vi "DAQ_olfactometer_control.vi"() -> ()   [LabVIEW 2016]
uses:
  <vilib>/DAQmx/write.llb/DAQmx Write (Digital 1D Wfm NChan NSamp).vi
  <vilib>/DAQmx/read.llb/DAQmx Read (Analog 1D Wfm NChan NSamp).vi
  <vilib>/Waveform/DWDTOps.llb/DWDT Uncompress Digital.vi
  <vilib>/DAQmx/miscellaneous.llb/DAQmx Fill In Error Info.vi
panel:
  out "flows":waveform(dbl)[](graph)
  in  "Analog input sampling time (s)":dbl=2.0 format="%#_13g"
  in  "Odour bottles":T1(array[cluster])=[[{"Mixture components"=[{"Name"="MINERAL OIL", "CID"=0, "Volatility"=0.0}], "Name"="B1 (Bl)", "VPs"="0.0E+0", "Proportion"=[{"Numeric"=100.0}], "Selected"=FALSE, "Counter"=TRUE}, {"Mixture components"=[{"Name"="Methyl benzoate", "CID"=8103, "Volatility"=0.38}, {"Name"="Menthone", "CID"=8063, "Volatility"=0.28}], "Name"="B3 (ME2)", "VPs"="3.3E-1 ± 21%", "Proportion"=[{"Numeric"=50.0}, {"Numeric"=50.0}], "Selected"=TRUE, "Counter"=FALSE}, {"Mixture components"=[{"Name"="Decanol", "CID"=460, "Volatility"=0.00851}], "Name"="B5 (C4f)", "VPs"="8.5E-3", "Proportion"=[{"Numeric"=100.0}], "Selected"=FALSE, "Counter"=FALSE}, {"Mixture components"=[{"Name"="Acetophenone", "CID"=8174, "Volatility"=0.45}, {"Name"="Fenchone", "CID"=8635, "Volatility"=0.82}], "Name"="B7 (ME1)", "VPs"="6.4E-1 ± 41%", "Proportion"=[{"Numeric"=50.0}, {"Numeric"=50.0}], "Selected"=FALSE, "Counter"=FALSE}], [{"Mixture components"=[{"Name"="MINERAL OIL", "CID"=0, "Volatility"=0.0}], "Name"="B2 (Bl)", "VPs"="0.0E+0", "Proportion"=[{"Numeric"=100.0}], "Selected"=FALSE, "Counter"=TRUE}, {"Mixture components"=[{"Name"="Octanol", "CID"=7439, "Volatility"=0.0794}], "Name"="B4 (C4cA)", "VPs"="7.9E-2", "Proportion"=[{"Numeric"=100.0}], "Selected"=FALSE, "Counter"=FALSE}, {"Mixture components"=[{"Name"="MINERAL OIL", "CID"=0, "Volatility"=0.0}], "Name"="B6 (Bl)", "VPs"="0.0E+0", "Proportion"=[{"Numeric"=100.0}], "Selected"=FALSE, "Counter"=FALSE}, {"Mixture components"=[{"Name"="Heptanoic acid ", "CID"=957, "Volatility"=0.0107}], "Name"="B8 (C3cA)", "VPs"="1.1E-2", "Proportion"=[{"Numeric"=100.0}], "Selected"=FALSE, "Counter"=FALSE}], [{"Mixture components"=[{"Name"="MINERAL OIL", "CID"=0, "Volatility"=0.0}], "Name"="B9 (Bl)", "VPs"="0.0E+0", "Proportion"=[{"Numeric"=100.0}], "Selected"=FALSE, "Counter"=TRUE}, {"Mixture components"=[{"Name"="Geranyl acetate", "CID"=6985, "Volatility"=0.03}, {"Name"="Dimethylacetophenone", "CID"=7144, "Volatility"=0.063}], "Name"="B11 (MW1)", "VPs"="4.6E-2 ± 50%", "Proportion"=[{"Numeric"=50.0}, {"Numeric"=50.0}], "Selected"=FALSE, "Counter"=FALSE}, {"Mixture components"=[{"Name"="Geraniol", "CID"=6405, "Volatility"=0.03}, {"Name"="Phenyl butanone", "CID"=7762, "Volatility"=0.1}], "Name"="B13 (MW2)", "VPs"="6.5E-2 ± 76%", "Proportion"=[{"Numeric"=50.0}, {"Numeric"=50.0}], "Selected"=FALSE, "Counter"=FALSE}, {"Mixture components"=[{"Name"="Methylheptanoic acid", "CID"=1032, "Volatility"=0.018}], "Name"="B15 (C3f)", "VPs"="1.8E-2", "Proportion"=[{"Numeric"=100.0}], "Selected"=FALSE, "Counter"=FALSE}], [{"Mixture components"=[{"Name"="MINERAL OIL", "CID"=0, "Volatility"=0.0}], "Name"="B10 (Bl)", "VPs"="0.0E+0", "Proportion"=[{"Numeric"=100.0}], "Selected"=FALSE, "Counter"=FALSE}, {"Mixture components"=[{"Name"="Valeric acid", "CID"=8025, "Volatility"=0.196}], "Name"="B12 (C3cB)", "VPs"="2.0E-1", "Proportion"=[{"Numeric"=100.0}], "Selected"=FALSE, "Counter"=FALSE}, {"Mixture components"=[{"Name"="Nonanol", "CID"=4133, "Volatility"=0.0227}], "Name"="B14 (C4cB)", "VPs"="2.3E-2", "Proportion"=[{"Numeric"=100.0}], "Selected"=FALSE, "Counter"=FALSE}, {"Mixture components"=[{"Name"="Hydroxacetophenone", "CID"=7462, "Volatility"=0.0856}], "Name"="B16 (Ol)", "VPs"="8.6E-2", "Proportion"=[{"Numeric"=100.0}], "Selected"=FALSE, "Counter"=FALSE}]]
  in  "Olfactometer parameters":T2={"Back valve ON delays"=[0.0, 0.0, 0.0, 0.0, 0.0, 0.0, 0.0, 0.0, 0.0, 0.0, 0.0, 0.0, 0.0, 0.0, 0.0, 0.0], "Back valve OFF delays"=[0.0, 0.0, 0.0, 0.0, 0.0, 0.0, 0.0, 0.0, 0.0, 0.0, 0.0, 0.0, 0.0, 0.0, 0.0, 0.0], "Step duration (ms)"=2.0, "TTL binary step duration (ms)"=1.0, "Sampling rate (Hz)"=20000.0, "Initial delay (ms)"=0.0, "Pulse duration (ms)"=250.0} {"Initial delay (ms)" format="%#_13g"}
  in  "Stimulus parameters":T3={"Name"="", "Active bottles"=[3, 6], "Concentrations"=[1.0], "Unit"=enum."ppm"}
  out "error out":errorcluster
  in  "error in":errorcluster
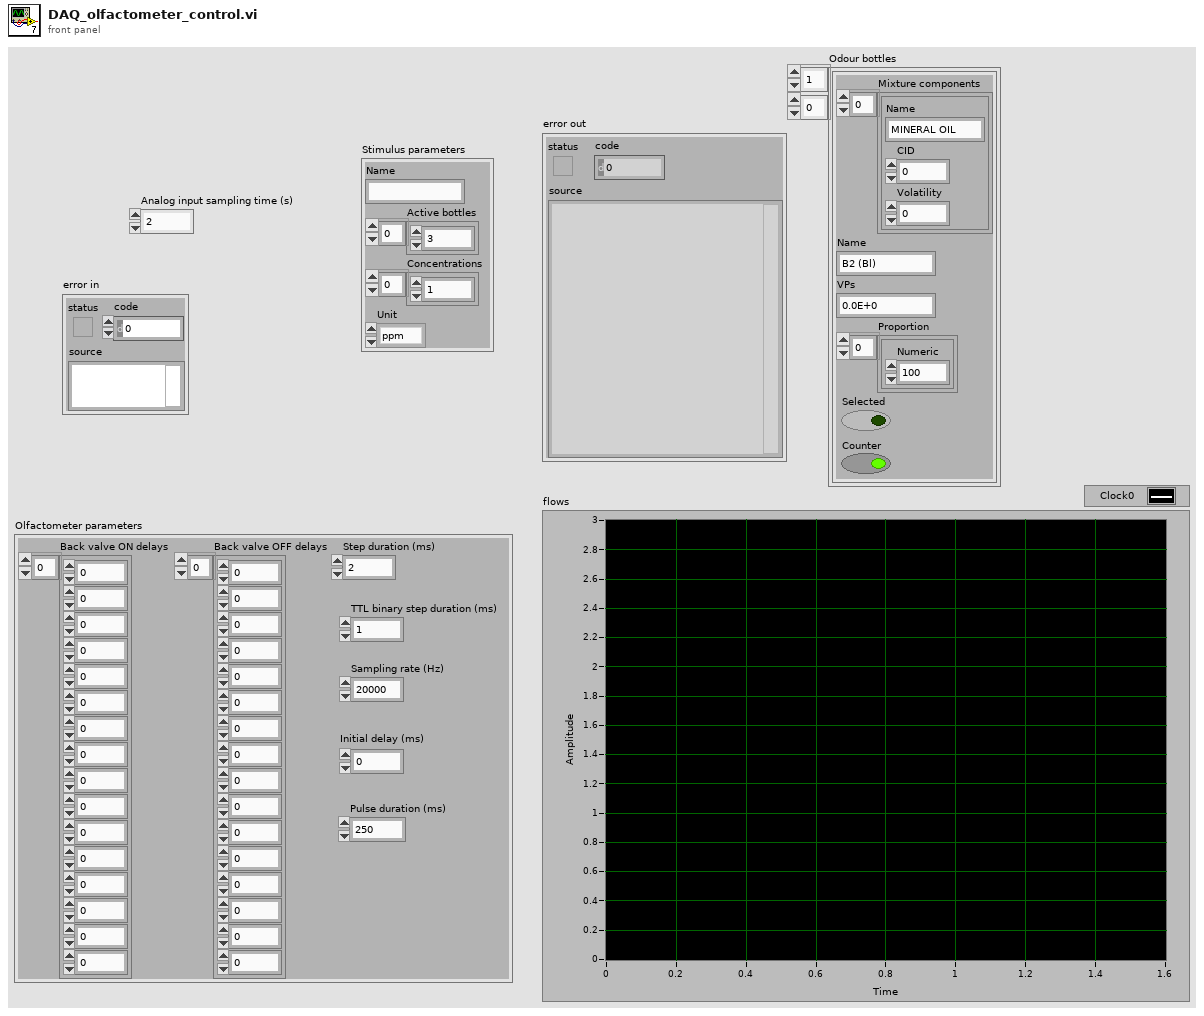
[diagram p1: front panel]
types:
  T1 = cluster{"Mixture components":cluster{"Name":string, "CID":i32, "Volatility":dbl}[], "Name":string, "VPs":string, "Proportion":cluster{"Numeric":dbl}[], "Selected":bool, "Counter":bool}[][]
  T2 = cluster{"Back valve ON delays":dbl[], "Back valve OFF delays":dbl[], "Step duration (ms)":dbl, "TTL binary step duration (ms)":dbl, "Sampling rate (Hz)":dbl, "Initial delay (ms)":dbl, "Pulse duration (ms)":dbl}
  T3 = cluster{"Name":string, "Active bottles":i32[], "Concentrations":dbl[], "Unit":enum16{"%", "ppm"}}
  T4 = cluster{"Name":string, "Active bottles":i32[], "Concentrations":dbl[], "Unit":enum16{"%", "ppm"}, "Pulse duration (ms)":dbl}
  T5 = typedef "NI_cluster.ctl" = refnum<k21>
  T6 = cluster{"AI task out":refnum<k21>, "DO task out":T5, "AI samples":i32}
  T7 = cluster{"VISA Refnum in":refnum<visa-resource-name>, "error in (no error)":errorcluster}
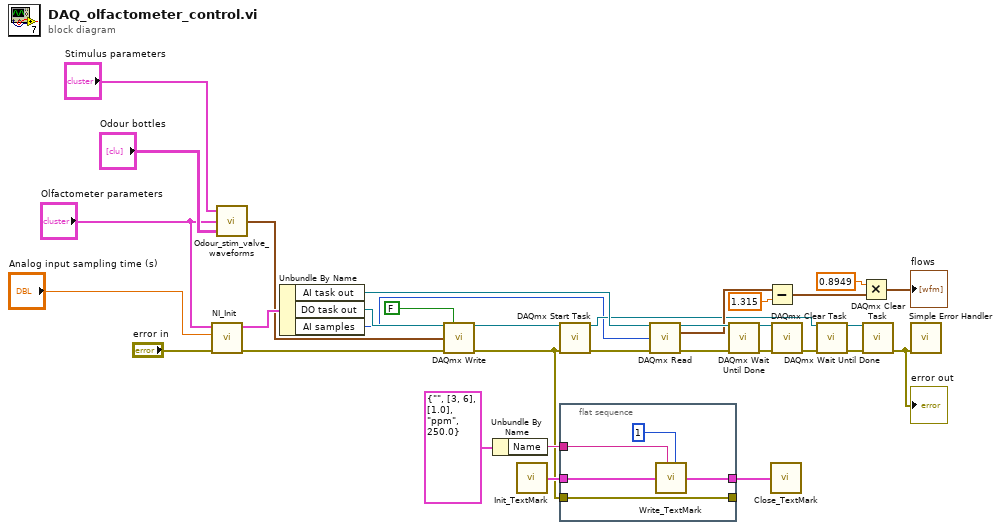
[diagram p0: block diagram]
diagram:
  n1 = call "NI_Init.vi"("error in (no error)"="error in", "Analog input sampling time (s)"="Analog input sampling time (s)", "Olfactometer parameters"="Olfactometer parameters") -> ("error out"=w3:errorcluster, "NI cluster out"=w22:T6)  [unwired: 4 in]
  n2 = call "Odour_stim_valve_waveforms.vi"("Odour bottles"="Odour bottles", "Olfactormeter parameters"="Olfactometer parameters", "Stimulus parameters"="Stimulus parameters") -> ("waveform array"=w14:digitalwaveform[])
  n3 = Unbundle By Name(w22) -> ("AI task out"=w21:refnum<k21>, "DO task out"=w4:T5, "AI samples"=w1:i32)
  n4 = call-poly <vilib>:"DAQmx Write.vi"("task/channels in"=w4, "auto start"=FALSE, "data"=w14, "error in"=w3) -> ("task out"=w13:refnum<k21>, "error out"=w2:errorcluster)  [unwired: 9 in, 1 out]
  n5 = Unbundle By Name(T4 {"Name"="", "Active bottles"=[3, 6], "Concentrations"=[1.0], "Unit"=enum."ppm", "Pulse duration (ms)"=250.0} ("Stimulus parameters")) -> ("Name"=w27:string)
  n6 = call "Init_TextMark.vi"() -> ("TextMark out"=w29:T7)
  n7 = call <vilib>:"DAQmx Start Task.vi"("task/channels in"=w13, "error in"=w2) -> ("task out"=w10:refnum<k21>, "error out"=w9:errorcluster)  [unwired: 12 in]
  n8 = flat-sequence {
    tunnel: w29 -> [w38]
    tunnel: [w37] -> w28
    tunnel: w27 -> [w36]
    tunnel: [w34] -> _
    tunnel: w2 -> [w34]
    frame #0 {
      n9 = call "Write_TextMark.vi"("text"=w36, "TextMark in"=w38, "type"=1) -> ("TextMark out"=w37:T7)  [unwired: 6 in]
    }
  }
  n10 = call-poly <vilib>:"DAQmx Read.vi"("task/channels in"=w21, "number of samples per channel"=w1, "error in"=w9) -> ("task out"=w31:refnum<k21>, "data"=w17:waveform(dbl)[], "error out"=w7:errorcluster)  [unwired: 10 in]
  n11 = call <vilib>:"DAQmx Wait Until Done.vi"("task/channels in"=w31, "error in"=w7) -> ("task out"=w12:refnum<k21>, "error out"=w11:errorcluster)  [unwired: 12 in]
  n12 = Subtract(x=w17, y=1.315) -> (x-y=w18:waveform(dbl)[])
  n13 = call "Close_TextMark.vi"("TextMark in"=w28) -> ()
  n14 = call <vilib>:"DAQmx Clear Task.vi"("task in"=w12, "error in"=w11) -> ("error out"=w6:errorcluster)  [unwired: 13 in]
  n15 = call <vilib>:"DAQmx Wait Until Done.vi"("task/channels in"=w10, "error in"=w6) -> ("task out"=w8:refnum<k21>, "error out"=w5:errorcluster)  [unwired: 12 in]
  n16 = Multiply(x=0.8949, y=w18) -> (x*y=→"flows":waveform(dbl)[])
  n17 = call <vilib>:"DAQmx Clear Task.vi"("task in"=w8, "error in"=w5) -> ("error out"=w32:errorcluster)  [unwired: 13 in]
  "error out" <- w32
  n18 = call <vilib>:"Simple Error Handler.vi"("error in (no error)"=w32) -> ()  [unwired: 4 in, 5 out]
